vi "MPU_Stick_3D_View_Updater.vi"(8 "error in (no error)":errorcluster, 11 "MPU_Stick_Globals":T1) -> ()   [LabVIEW 2017]
uses:
  Controls/MPU_Stick_Globals.ctl
  Controls/IMU_Configuration_References.ctl
  Controls/MP_Comp_Filter_Constants_References.ctl
  Controls/MD_Threshold_References.ctl
  Controls/MD_Type_References.ctl
  Controls/LED_Configuration_References.ctl
  Controls/Primary_References.ctl
  Controls/MPU_Stick_Queues.ctl
  Controls/MPU_Stick_Queue_Element.ctl
  Controls/MPU_Stick_Queue_Commands.ctl
  Classes/ADCP.lvclass
  Controls/MPU_Stick_Timestamped_Data.ctl
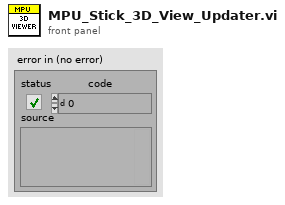
[diagram p1: front panel]
types:
  T1 = typedef "MPU_Stick_Globals.ctl" = cluster{"IMU_configuration_references":T2, "MP_Comp_Filter_Constants_References":T3, "MD_Threshold_References":T4, "MD_Type_References":T5, "LED_Configuration_References":T6, "Primary_references":T7, "MPU_Stick_Queues":T8, "ADCP":refnum<vi>}
  T2 = typedef "IMU_Configuration_References.ctl" = cluster{"Get all IMU configurations":refnum<vi>, "Set all IMU configurations":refnum<vi>, "Get sampling frequency":refnum<vi>, "Set sampling frequency":refnum<vi>, "Get calibration point count":refnum<vi>, "Set calibration point count":refnum<vi>, "Get calibration interval":refnum<vi>, "Set calibration interval":refnum<vi>, "Get Gyroscope bandwidth":refnum<vi>, "Set Gyroscope bandwidth":refnum<vi>, "Get Gyroscope F.S. Value":refnum<vi>, "Set Gyroscope F.S. Value":refnum<vi>, "Get Accelerometer bandwidth":refnum<vi>, "Set Accelerometer bandwidth":refnum<vi>, "Get Accelerometer F.S. Value":refnum<vi>, "Set Accelerometer F.S. Value":refnum<vi>, "Sampling frequency (Hz)":refnum<vi>, "Calibration point count":refnum<vi>, "Calibration interval (ms)":refnum<vi>, "IMU Gyroscope bandwidth":refnum<vi>, "IMU Gyroscope F.S. value":refnum<vi>, "IMU Accelerometer bandwidth":refnum<vi>, "IMU Accelerometer F.S. value":refnum<vi>}
  T3 = typedef "MP_Comp_Filter_Constants_References.ctl" = cluster{"Set pitch filter constant":refnum<vi>, "Get pitch filter constant":refnum<vi>, "Set roll filter constant":refnum<vi>, "Get roll filter constant":refnum<vi>, "Pitch filter constant":refnum<vi>, "Roll filter constant":refnum<vi>}
  T4 = typedef "MD_Threshold_References.ctl" = cluster{"Yaw threshold (U)":refnum<vi>, "Yaw threshold (L)":refnum<vi>, "Pitch threshold (U)":refnum<vi>, "Pitch. threshold (L)":refnum<vi>, "Roll threshold (U)":refnum<vi>, "Roll threshold (L)":refnum<vi>, "Z gyro. threshold (U)":refnum<vi>, "Z gyro. threshold (L)":refnum<vi>, "Y gyro. threshold (U)":refnum<vi>, "Y gyro. threshold (L)":refnum<vi>, "X gyro. threshold (U)":refnum<vi>, "X gyro. threshold (L)":refnum<vi>, "Z accel. threshold (U)":refnum<vi>, "Z accel. threshold (L)":refnum<vi>, "Y accel. threshold (U)":refnum<vi>, "Y accel. threshold (L)":refnum<vi>, "X accel. threshold (U)":refnum<vi>, "X accel. threshold (L)":refnum<vi>, "Set all Motion detection threshold configurations":refnum<vi>, "Get yaw threshold (upper)":refnum<vi>, "Get yaw threshold (lower)":refnum<vi>, "Get pitch threshold (upper)":refnum<vi>, "Get pitch threshold (lower)":refnum<vi>, "Get roll threshold (upper)":refnum<vi>, "Get roll threshold (lower)":refnum<vi>, "Get Z gyro threshold (upper)":refnum<vi>, "Get Z gyro threshold (lower)":refnum<vi>, "Get Y gyro threshold (upper)":refnum<vi>, "Get Y gyro threshold (lower)":refnum<vi>, "Get X gyro threshold (upper)":refnum<vi>, "Get X gyro threshold (lower)":refnum<vi>, "Get Z accel threshold (upper)":refnum<vi>, "Get Z accel threshold (lower)":refnum<vi>, "Get Y accel threshold (upper)":refnum<vi>, "Get Y accel threshold (lower)":refnum<vi>, "Get X accel threshold (upper)":refnum<vi>, "Get X accel threshold (lower)":refnum<vi>, "Get all Motion detection threshold configurations":refnum<vi>, "Set yaw threshold (upper)":refnum<vi>, "Set yaw threshold (lower)":refnum<vi>, "Set pitch threshold (upper)":refnum<vi>, "Set pitch threshold (lower)":refnum<vi>, "Set roll threshold (upper)":refnum<vi>, "Set roll threshold (lower)":refnum<vi>, "Set Z gyro threshold (upper)":refnum<vi>, "Set Z gyro threshold (lower)":refnum<vi>, "Set Y gyro threshold (upper)":refnum<vi>, "Set Y gyro threshold (lower)":refnum<vi>, "Set X gyro threshold (upper)":refnum<vi>, "Set X gyro threshold (lower)":refnum<vi>, "Set Z accel threshold (upper)":refnum<vi>, "Set Z accel threshold (lower)":refnum<vi>, "Set Y accel threshold (upper)":refnum<vi>, "Set Y accel threshold (lower)":refnum<vi>, "Set X accel threshold (upper)":refnum<vi>, "Set X accel threshold (lower)":refnum<vi>}
  T5 = typedef "MD_Type_References.ctl" = cluster{"Yaw threshold type":refnum<vi>, "Pitch threshold type":refnum<vi>, "Roll threshold type":refnum<vi>, "Z gyro threshold type":refnum<vi>, "Y gyro threshold type":refnum<vi>, "X gyro threshold type":refnum<vi>, "Z accel threshold type":refnum<vi>, "Y accel threshold type":refnum<vi>, "X accel threshold type":refnum<vi>, "Set all Motion detection type configurations":refnum<vi>, "Get all Motion detection type configurations":refnum<vi>, "Set yaw threshold type":refnum<vi>, "Get yaw threshold type":refnum<vi>, "Set pitch threshold type":refnum<vi>, "Get pitch threshold type":refnum<vi>, "Set roll threshold type":refnum<vi>, "Get roll threshold type":refnum<vi>, "Set Z gyroscope threshold type":refnum<vi>, "Get Z gyroscope threshold type":refnum<vi>, "Set Y gyroscope threshold type":refnum<vi>, "Get Y gyroscope threshold type":refnum<vi>, "Set X gyroscope threshold type":refnum<vi>, "Get X gyroscope threshold type":refnum<vi>, "Set Z accel threshold type":refnum<vi>, "Get Z accel threshold type":refnum<vi>, "Set Y accel threshold type":refnum<vi>, "Get Y accel threshold type":refnum<vi>, "Get X accel threshold type":refnum<vi>, "Set X accel threshold type":refnum<vi>}
  T6 = typedef "LED_Configuration_References.ctl" = cluster{"Get all LED configurations":refnum<vi>, "Set all LED configurations":refnum<vi>, "Get LED3 configuration":refnum<vi>, "Set LED3 configuration":refnum<vi>, "Get LED2 configuration":refnum<vi>, "Set LED2 configuration":refnum<vi>, "Get LED1 configuration":refnum<vi>, "Set LED1 configuration":refnum<vi>, "LED3 Configuration":refnum<vi>, "LED2 Configuration":refnum<vi>, "LED1 Configuration":refnum<vi>}
  T7 = typedef "Primary_References.ctl" = cluster{"3D View Image":refnum<vi>, "Plot":refnum<vi>, "Graph / 3D view tab control":refnum<vi>, "MP Reset":refnum<vi>, "Calibrate IMU":refnum<vi>, "Plot Parameter List":refnum<vi>, "Remove Parameter from Plot":refnum<vi>, "Add Parameter to Plot":refnum<vi>, "Parameter to monitor":refnum<vi>, "Yaw motion detection output":refnum<vi>, "Pitch motion detection output":refnum<vi>, "Roll motion detection output":refnum<vi>, "Z gyro motion detection output":refnum<vi>, "Y gyro motion detection output":refnum<vi>, "X gyro motion detection output":refnum<vi>, "Z accel motion detection output":refnum<vi>, "Y accel motion detection output":refnum<vi>, "X accel motion detection output":refnum<vi>, "Yaw angle (filter) (degrees)":refnum<vi>, "Pitch angle (filter) (degrees)":refnum<vi>, "Roll angle (filter) (degrees)":refnum<vi>, "Yaw angle (gyro) (degrees)":refnum<vi>, "Pitch angle (gyro) (degrees)":refnum<vi>, "Roll angle (gyro) (degrees)":refnum<vi>, "Yaw angle (accel) (degrees)":refnum<vi>, "Pitch angle (accel) (degrees)":refnum<vi>, "Roll angle (accel) (degrees)":refnum<vi>, "Z gyroscope reading (DPS)":refnum<vi>, "Y gyroscope reading (DPS)":refnum<vi>, "X gyroscope reading (DPS)":refnum<vi>, "Z accelerometer reading (G)":refnum<vi>, "Y accelerometer reading (G)":refnum<vi>, "X accelerometer reading (G)":refnum<vi>, "Save all config.":refnum<vi>, "Write all config.":refnum<vi>, "Read all config.":refnum<vi>, "Tab Control":refnum<vi>, "Baud Rate":refnum<vi>, "COM Port":refnum<vi>, "Time (ms)":refnum<vi>, "Value (Units)":refnum<vi>, "Exit Application":refnum<vi>, "Connect Device":refnum<vi>, "Progress Bar":refnum<vi>, "Get Range & Offset":refnum<vi>, "Range":refnum<vi>, "Offset":refnum<vi>, "Set Range & Offset":refnum<vi>, "Parameter name":refnum<vi>, "Plot time (ms)":refnum<vi>, "Plot value":refnum<vi>}
  T8 = typedef "MPU_Stick_Queues.ctl" = cluster{"UI Event Handler":refnum<queue>, "3D View Updater":refnum<queue>, "Plot Updater":refnum<queue>, "Serial Port Reader":refnum<queue>, "UI Indicators Updater":refnum<queue>}
  T9 = typedef "MPU_Stick_Timestamped_Data.ctl" = cluster{"Parameter name":string, "Time (ms)":dbl, "Value":dbl}
  T10 = typedef "MPU_Stick_Queue_Element.ctl" = cluster{"Data":variant, "Command":T11}
  T11 = typedef "MPU_Stick_Queue_Commands.ctl" = enum16{"UI_Event_Exit_Application_RQST", "UI_Event_Exit_Application_ACK", "UI_Event_Connect_Device_RQST", "UI_Event_Connect_Device_ACK", "UI_Event_Disconnect_Device_RQST", "UI_Event_Disconnect_Device_ACK", "UI_Event_Read_All_Configurations_RQST", "UI_Event_Read_All_Configurations_ACK", "UI_Event_Write_All_Configurations_RQST", "UI_Event_Write_All_Configurations_ACK", "UI_Event_Save_All_Configurations_RQST", "UI_Event_Save_All_Configurations_ACK", "UI_Event_Calibrate_IMU_Sensor_RQST", "UI_Event_Calibrate_IMU_Sensor_ACK", "UI_Event_MP_Reset_RQST", "UI_Event_MP_Reset_ACK", "UI_Event_Get_Config_RQST", "UI_Event_Get_Config_ACK", "UI_Event_Set_Config_RQST", "UI_Event_Set_Config_ACK", "Read_Serial_Port_Data_Pause", "Read_Serial_Port_Data_Continue", "Read_Serial_Port_Data_Exit", "Plotter_Exit", "Plotter_Update", "Plotter_Add_Channel", "Plotter_Remove_Channel", "3D Viewer Update", "3D Viewer Exit", "UI Indicators Update", "UI Indicators Exit"}
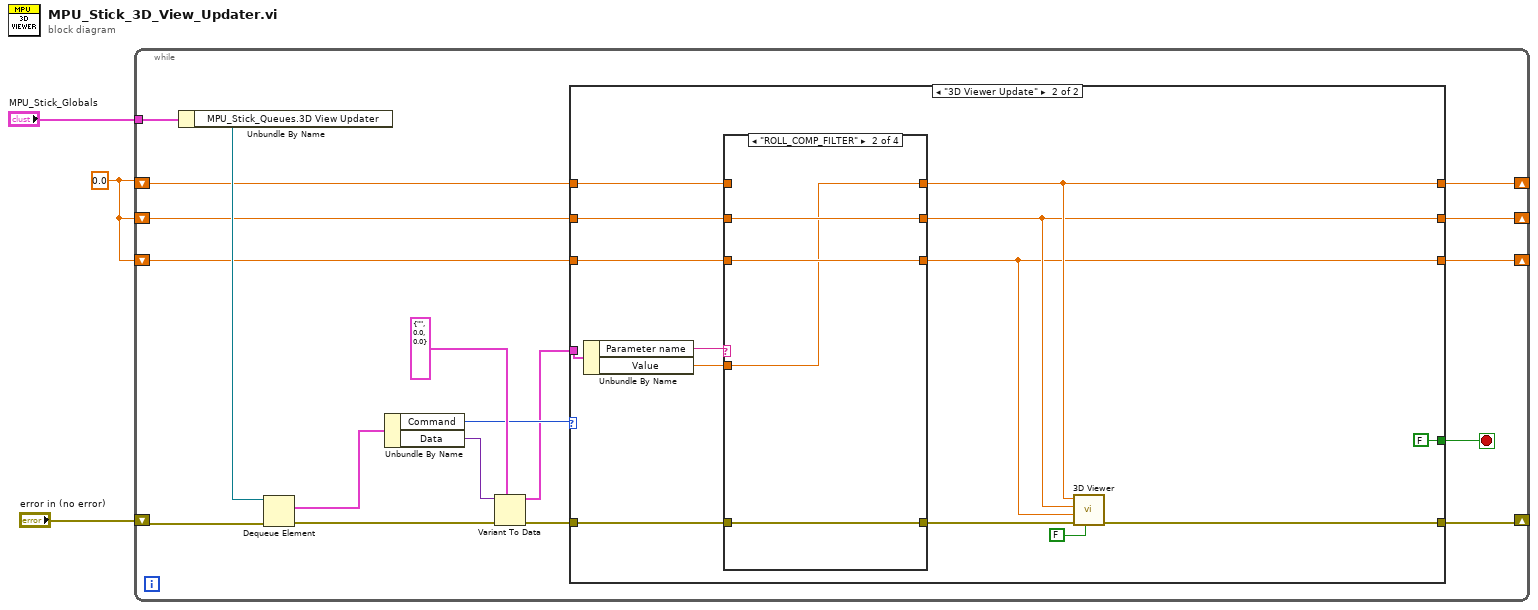
[diagram p0: block diagram]
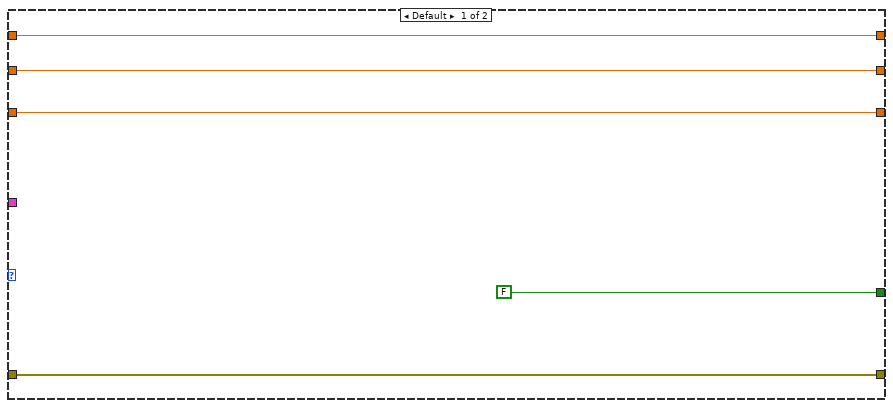
[diagram p2: hidden frame]
diagram:
  w1 = 0.0
  n1 = while {
    tunnel: "MPU_Stick_Globals" -> [w21]
    shift-right: [w12] -> _
    shift-left: "error in (no error)" -> [w20]
    shift-right: [w9] -> _
    shift-left: w1 -> [w10]
    shift-right: [w7] -> _
    shift-left: w1 -> [w8]
    shift-right: [w5] -> _
    shift-left: w1 -> [w6]
    stop <- w11 stop-if-true
    n2 = Unbundle By Name(w21) -> ("MPU_Stick_Queues.3D View Updater"=w19:refnum<queue>)
    n3 = Dequeue Element(queue=w19, error in (no error)=w20) -> (element=w18:T10, error out=w17:errorcluster)  [unwired: 1 in, 2 out]
    n4 = Unbundle By Name(w18) -> ("Command"=w14:T11, "Data"=w16:variant)
    n5 = Variant To Data(error in=w17, type=T9 {"Parameter name"="", "Time (ms)"=0.0, "Value"=0.0} ("Cluster"), Variant=w16) -> (data=w4:T9, error out=w13:errorcluster)
    n6 = case shown="\"3D Viewer Update\"" w14 {
      tunnel: w13 -> [w26 w39]
      tunnel: [w26 w31] -> w12
      tunnel: [FALSE FALSE] -> w11
      tunnel: w10 -> [w24 w36]
      tunnel: [w24 w29] -> w9
      tunnel: w8 -> [w23 w35]
      tunnel: [w23 w28] -> w7
      tunnel: w6 -> [w22 w34]
      tunnel: [w22 w27] -> w5
      tunnel: w4 -> [_ w38]
      frame Default {
      }
      frame "3D Viewer Update" {
        n7 = Unbundle By Name(w38) -> ("Parameter name"=w37:string, "Value"=w33:dbl)
        n8 = case shown="\"ROLL_COMP_FILTER\"" w37 {
          tunnel: w39 -> [w41 w45 w51 w56]
          tunnel: w36 -> [w44 _ w50 w55]
          tunnel: [w44 w46 w50 w55] -> w29
          tunnel: w35 -> [w43 w48 _ w54]
          tunnel: [w43 w48 w49 w54] -> w28
          tunnel: w34 -> [w42 w47 w52 _]
          tunnel: [w42 w47 w52 w53] -> w27
          tunnel: [w41 w45 w51 w56] -> w32
          tunnel: w33 -> [_ w46 w49 w53]
          frame Default {
          }
          frame "ROLL_COMP_FILTER" {
          }
          frame "PITCH_COMP_FILTER" {
          }
          frame "YAW_COMP_FILTER" {
          }
        }
        n9 = call "3D Viewer.vi"("Initialize ?"=FALSE, "error in (no error)"=w32, "Angle Z"=w27, "Angle Y"=w28, "Angle X"=w29) -> ("error out"=w31:errorcluster)  [unwired: 5 in, 1 out]
      }
    }
  }
